vi "Get Data.vi"(8 "error in":errorcluster, 11 "nCRD in":refnum<class "nCRD.lvclass">) -> (0 "error out":errorcluster, 3 "nCRD out":refnum<class "nCRD.lvclass">)   [LabVIEW 2015, in "nCRD.lvclass"]
doc: "Retrieve the data from the given cards. Set the <B>goodData</B> flag to True and log any errors that will be handled down the line. If there is an error associated with the collection of the data, the <B>goodData</B> flag will be set to false when the logged errors are handled.\nThe ringdown traces recorded in the <B>HF AI</B> task are divided up into a m x n matrix where:\n * m = YAG pulse rate\n * n = YAG duty cycle * HF AI Sampling Rate / YAG Pulse Rate"
uses:
  nCRD.lvclass
  Reusable/Instrument/state.ctl
  Session/Raw FPGA/FPGA Session.lvclass
  nCRD.lvclass/nCRD.ctl
  Session/Raw FPGA/FPGA Session.lvclass/FPGA Session.ctl
  Reusable/CRDS/Main/CRDS.lvclass/CRDS.ctl
  Session/Raw FPGA/Read FPGA Ref.vi
  Reusable/CRDS/Main/Write Laser Data.vi
  Reusable/CRDS/Main/Read Data.vi
  <vilib>/Utility/error.llb/Error Cluster From Error Code.vi
  <vilib>/rvi/errors/niLvFpgaAdjustHostInterfaceError.vi
  Reusable/Data/Write measTime.vi
  Reusable/CRDS/Main/Write Data.vi
  Reusable/CRDS/Main/Write goodData.vi
  Reusable/CRDS/Data/Main/CRDS Data.lvclass
  FPGA Ref.ctl
  <vilib>/rvi/interface/nirviMethod/nirviMethod.xnode
  FPGA Bitfiles/NickIO.lvbitx
  Reusable/Instrument/Instrument.lvclass
  <vilib>/FPGAPlugInAG/cRIO-9081/niLvFpga_ReadFifo_cRIO-9081.vi
  <vilib>/rvi/errors/niLvFpgaMergeErrorWithErrorCode.vi
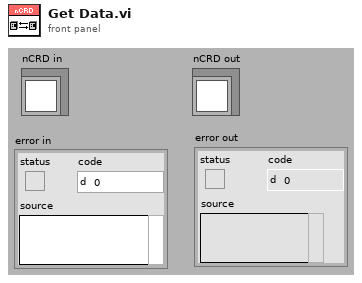
[diagram p1: front panel]
types:
  T1 = typedef "Instrument.lvclass/state.ctl" = enum8{"Configure", "Acquire", "Wait", "Quit", "Handle Error", "NOOP"}
  T2 = typedef "Session - Root.lvclass/Session Handle.ctl" = refnum<data-value>
  T3 = typedef "FPGA Ref.ctl" = refnum<k20>
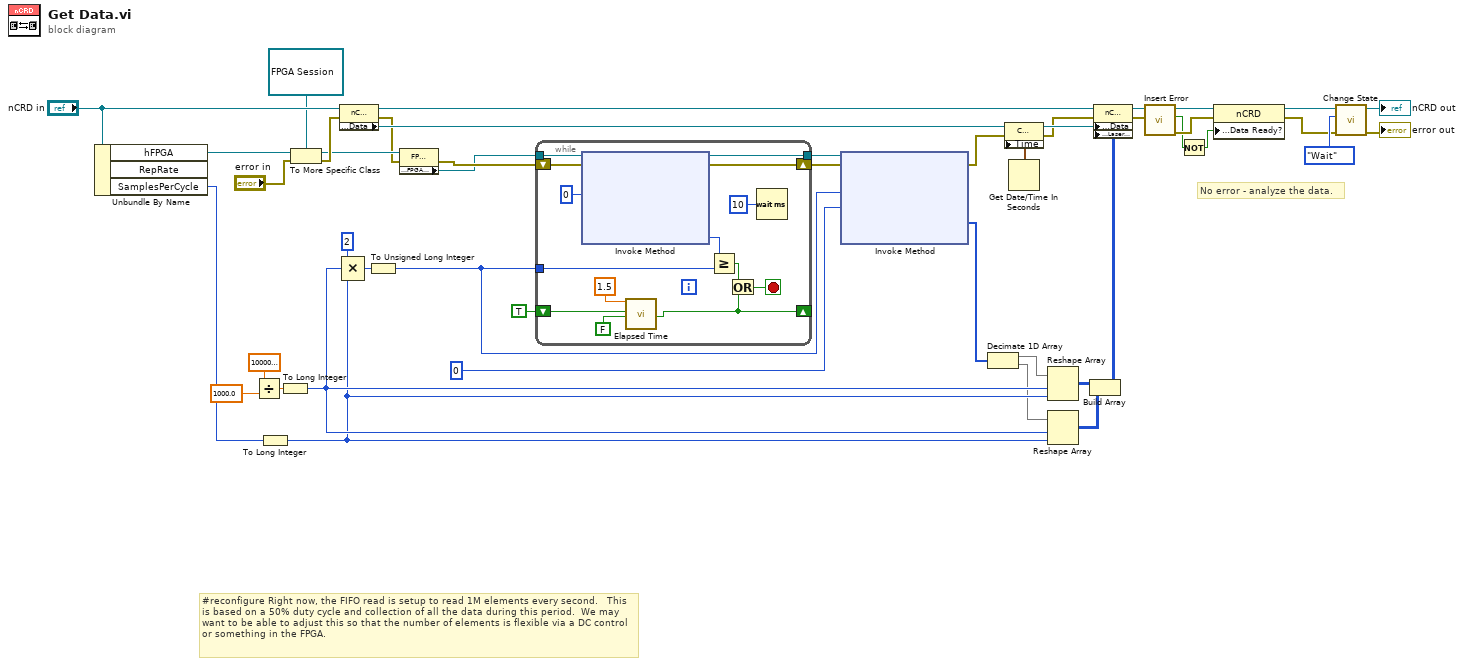
[diagram p0: block diagram]
diagram:
  # "No error - analyze the data."
  # "#reconfigure Right now, the FIFO read is setup to read 1M elements every second.   This is based on a 50% duty cycle and collection of all the data during this period.  We may want to be able to adjust this so that the number of elements is flexible via a DC control or something in the FPGA."
  n1 = Unbundle By Name("nCRD in") -> ("hFPGA"=w22:T2, "SamplesPerCycle"=w36:u16)  [unwired: 1 out]
  n2 = Divide(x=sgl 1000000.0, y=sgl 1000.0) -> (x/y=w38:sgl)
  n3 = To Long Integer(number=w36) -> (32bit integer=w35:i32)
  n4 = To Long Integer(number=w38) -> (32bit integer=w37:i32)
  n5 = To More Specific Class(target class=refnum<data-value> refnum ("hFPGA"), reference=w22, error in="error in") -> (specific class reference=w18:refnum<data-value>, error out=w19:errorcluster)
  n6 = property class="nCRD"(reference="nCRD in", error in=w19) -> (reference out=w28:refnum<class "nCRD.lvclass">, error out=w11:errorcluster, "Data Access:Data"=w26:refnum<class "CRDS Data.lvclass">)
  n7 = Compound Arithmetic op=MULTIPLY(2 ("value"), w37, w35) -> (w16:i32)
  n8 = To Unsigned Long Integer(number=w16) -> (unsigned 32bit integer=w5:u32)
  n9 = property class="FPGA Session"(reference=w18, error in=w11) -> (error out=w10:errorcluster, "Accessors:FPGA Ref"=w8:T3)  [unwired: 1 out]
  n10 = while {
    tunnel: w8 -> [w57]
    shift-right: [w58] -> w6
    shift-left: w10 -> [w59]
    tunnel: [w55] -> w7
    tunnel: w5 -> [w53]
    shift-right: [w49] -> _
    shift-left: TRUE ("Time has Elapsed") -> [w51]
    stop <- w48 stop-if-true
    n11 = xnode "Invoke Method"("FPGA VI Reference In"=w57, "error in"=w59, "Number of Elements"=u32 0) -> ("FPGA VI Reference Out"=w55:T3, "error out"=w58:errorcluster, "Elements Remaining"=w54:u32)  [unwired: 1 in, 1 out]
    n12 = call "Elapsed Time"("Time Target (s)"=1.5, "Reset"=w51, "Auto Reset"=FALSE) -> ("Time has Elapsed"=w49:bool)  [unwired: 9 in, 7 out]
    n13 = Greater Or Equal?(x=w54, y=w53) -> (x >= y?=w52:bool)
    n14 = Or(x=w52, y=w49) -> (x .or. y?=w48:bool)
    n15 = Wait (ms)(milliseconds to wait=u32 10) -> ()  [unwired: 1 out]
  }
  n16 = xnode "Invoke Method"("FPGA VI Reference In"=w7, "error in"=w6, "Number of Elements"=w5, "Timeout (ms)"=0) -> ("error out"=w3:errorcluster, "Data"=w1:i16[])  [unwired: 2 out]
  n17 = Decimate 1D Array(w1) -> (w14:i16[], w15:i16[])
  n18 = Get Date/Time In Seconds() -> (seconds since 1Jan1904=w25:timestamp)
  n19 = property class="CRDS"(reference=w26, error in=w3, "Time"=w25) -> (reference out=w24:refnum<class "CRDS Data.lvclass">, error out=w23:errorcluster)
  n20 = Reshape Array(w14, w37, w35) -> (w13:i16[][])
  n21 = Reshape Array(w15, w37, w35) -> (w12:i16[][])
  n22 = Build Array(w13, w12) -> (w27:i16[][][])
  n23 = property class="nCRD"(reference=w28, error in=w23, "Data Access:Data"=w24, "Data Access:Laser Data"=w27) -> (reference out=w34:refnum<class "nCRD.lvclass">, error out=w33:errorcluster)
  n24 = call "Insert Error.vi"("err"=w33, "Instrument in"=w34) -> ("error out"=w31:errorcluster, "error?"=w30:bool, "Instrument out"=w32:refnum<class "nCRD.lvclass">)  [unwired: 7 in]
  n25 = Not(x=w30) -> (.not. x?=w29:bool)
  n26 = property class="nCRD"(reference=w32, error in=w31, "Data Access:Data Ready?"=w29) -> (reference out=w42:refnum<class "nCRD.lvclass">, error out=w41:errorcluster)
  n27 = call "Change State.vi"("error in"=w41, "instr state"=state."Wait", "Instrument in"=w42) -> ("error out"=→"error out":errorcluster, "Instrument out"=→"nCRD out":refnum<class "nCRD.lvclass">)  [unwired: 7 in]
